vi "Adjust Dashboard Window_NO_RESIZE.vi"(6 "Sizing Refnums":T1, 9 "Size Constraints":cluster{"min tab width":i32, "w/h":dbl}, 10 "VI":refnum<vi>, 11 "WIn Mode":refnum<notifier>) -> ()   [LabVIEW 2023]
panel:
  in  "Str Refnum":refnum<vi>
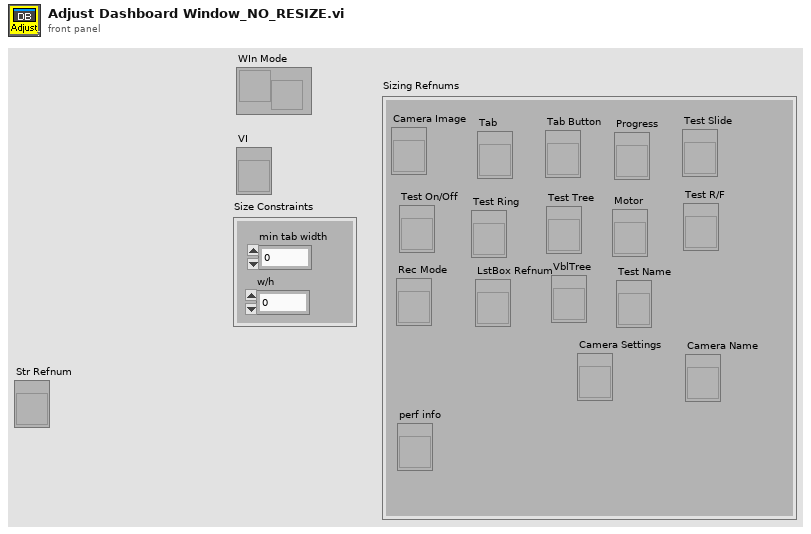
[diagram p1: front panel]
types:
  T1 = cluster{"Camera Image":refnum<vi>, "Tab":refnum<vi>, "Tab Button":refnum<vi>, "Rec Mode":refnum<vi>, "Test Slide":refnum<vi>, "Test On/Off":refnum<vi>, "Test Ring":refnum<vi>, "Test R/F":refnum<vi>, "Test Name":refnum<vi>, "Motor":refnum<vi>, "Progress":refnum<vi>, "LstBox Refnum":refnum<vi>, "Test Tree":refnum<vi>, "VblTree":refnum<vi>, "Camera Settings":refnum<vi>, "Camera Name":refnum<vi>, "perf info":refnum<vi>}
  T2 = typedef "LVRectTypeDef.ctl" = cluster{"Left":i16, "Top":i16, "Right":i16, "Bottom":i16}
  T3 = typedef "LVPointTypeDef.ctl" = cluster{"Horizontal":i16, "Vertical":i16}
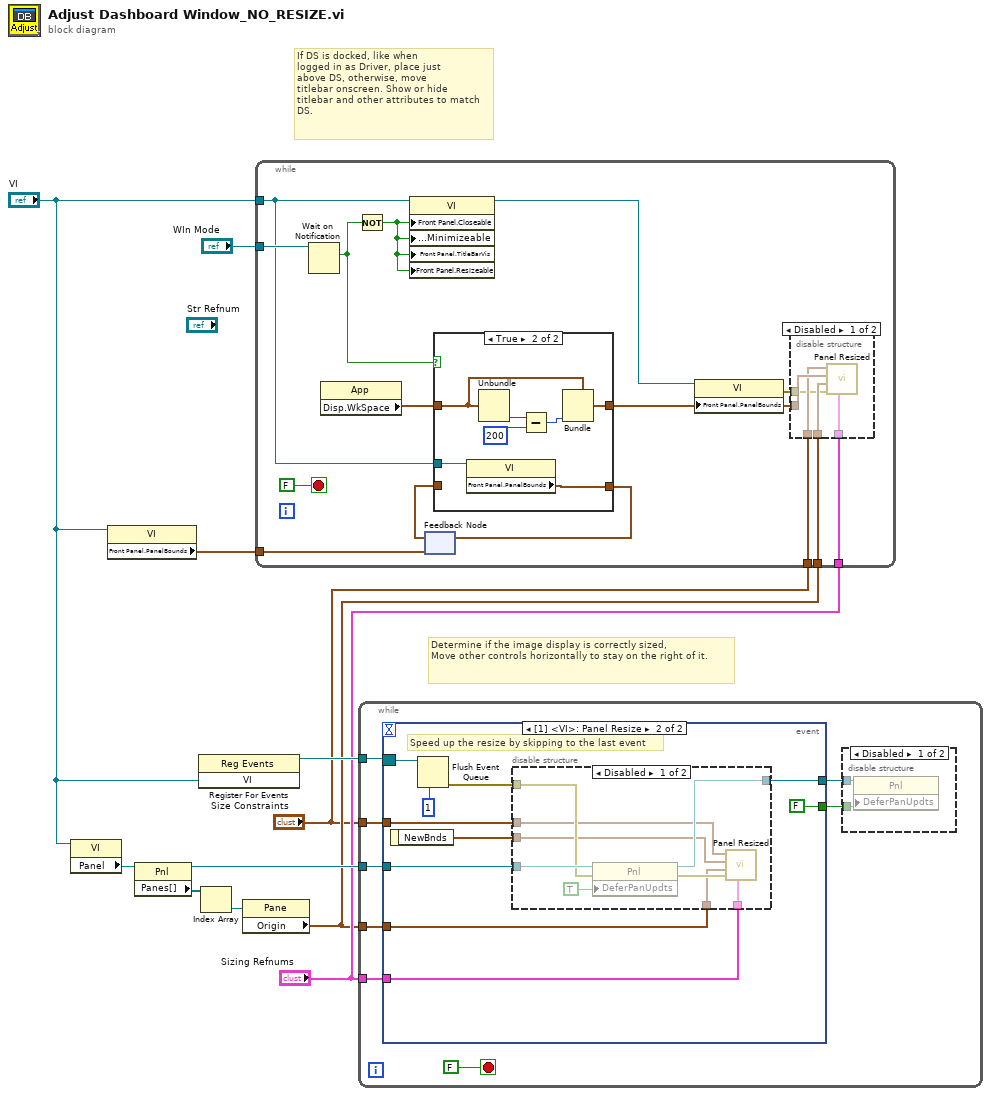
[diagram p0: block diagram]
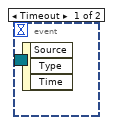
[diagram p3: hidden frame]
diagram:
  # "Determine if the image display is correctly sized,\nMove other controls horizontally to stay on the right of it."
  # "If DS is docked, like when\nlogged in as Driver, place just\nabove DS, otherwise, move\ntitlebar onscreen. Show or hide\ntitlebar and other attributes to match\nDS."
  n1 = property class="VI"(reference="VI") -> ("Panel"=w9:refnum<vi>)  [unwired: 1 in, 2 out]
  n2 = property class="VI"(reference="VI") -> ("Front Panel.PanelBounds"=w2:T2)  [unwired: 1 in, 2 out]
  n3 = property class="Pnl"(reference=w9) -> (reference out=w6:refnum<vi>, "Panes[]"=w8:refnum<vi>[])  [unwired: 1 in, 1 out]
  n4 = register-events("VI") -> (reference out=w10:refnum<event-registration>)  [unwired: 2 in, 1 out]
  n5 = Index Array(array=w8) -> (element=w7:refnum<vi>)  [unwired: 1 in]
  n6 = property class="Pane"(reference=w7) -> ("Origin"=w4:T3)  [unwired: 1 in, 2 out]
  n7 = while {
    tunnel: "WIn Mode" -> [w25]
    tunnel: "VI" -> [w17]
    tunnel: "Sizing Refnums" -> [w22]
    tunnel: w4 -> [w21]
    tunnel: "Size Constraints" -> [w19]
    tunnel: w2 -> [w14]
    stop <- FALSE stop-if-true
    n8 = Wait on Notification(notifier=w25) -> (notification=w18:bool)  [unwired: 3 in, 3 out]
    n9 = property class="App"() -> ("Disp.WkSpace"=w24:T2)  [unwired: 2 in, 2 out]
    n10 = Not(x=w18) -> (.not. x?=w13:bool)
    n11 = property class="VI"(reference=w17, "Front Panel.Closeable"=w13, "Front Panel.Minimizeable"=w13, "Front Panel.TitleBarVis"=w13, "Front Panel.Resizeable"=w13) -> (reference out=w23:refnum<vi>)  [unwired: 1 in, 1 out]
    n12 = feedback #1(w14) -> (w15:T2)
    n13 = case shown="True" w18 {
      tunnel: w24 -> [_ w35]
      tunnel: [w32 w36] -> w20
      tunnel: w17 -> [_ w34]
      tunnel: [w32 w33] -> w16
      tunnel: w15 -> [w32 _]
      frame False {
      }
      frame True {
        n14 = property class="VI"(reference=w34) -> ("Front Panel.PanelBounds"=w33:T2)  [unwired: 1 in, 2 out]
        n15 = Unbundle(w35) -> ("Bottom"=w39:i16)  [unwired: 3 out]
        n16 = Subtract(x=w39, y=200) -> (x-y=w37:i32)
        n17 = Bundle(cluster=w35, "Bottom"=w37) -> (w36:T2)  [unwired: 3 out]
      }
    }
    n18 = feedback-in #1(w16) -> ()
    n19 = property class="VI"(reference=w23, "Front Panel.PanelBounds"=w20) -> (error out=w12:errorcluster)  [unwired: 1 in, 1 out]
    n20 = disable-structure shown="Disabled" {
      disable-tunnel: w22 -> [w31 _]
      disable-tunnel: w21 -> [w30 _]
      disable-tunnel: w20 -> [w29 _]
      disable-tunnel: w19 -> [w28 _]
      disable-tunnel: w12 -> [w27 _]
      frame Disabled {
        n21 = call "Panel Resized.vi"("Sizing Refnums"=w31, "error in (no error)"=w27, "Origin"=w30, "NewBnds"=w29, "Size Constraints"=w28) -> ()  [unwired: 6 in, 1 out]
      }
      frame Enabled {
      }
    }
  }
  n22 = while {
    tunnel: w10 -> [w46]
    tunnel: "Sizing Refnums" -> [w45]
    tunnel: "Size Constraints" -> [w44]
    tunnel: w4 -> [w43]
    tunnel: w6 -> [w42]
    stop <- FALSE stop-if-true
    n23 = event shown="[1] <VI>: Panel Resize" {
      selector: w46 -> [_ w57]
      dyn-events: _ -> [_ _]
      timeout: _ -> [_ _]
      tunnel: w45 -> [_ w50]
      tunnel: w44 -> [_ w53]
      tunnel: w43 -> [_ w51]
      tunnel: w42 -> [_ w59]
      tunnel: [_ FALSE ("Defer Panel Updates")] -> w41
      tunnel: [_ w54] -> w40
      event Timeout {
        n24 = event-data() -> ()  [unwired: 1 in, 3 out]
      }
      event Panel Resize {
        # "Speed up the resize by skipping to the last event"
        n25 = event-data() -> ("NewBnds"=w52:T2)  [unwired: 1 in]
        n26 = Flush Event Queue(0:w57, 5:1 ("keep most recent")) -> (11:w55:errorcluster)  [unwired: 4 in, 2 out]
        n27 = disable-structure shown="Disabled" {
          disable-tunnel: w59 -> [w68 _]
          disable-tunnel: w55 -> [w66 _]
          disable-tunnel: [w65 _] -> w54
          disable-tunnel: w53 -> [w63 _]
          disable-tunnel: w52 -> [w62 _]
          disable-tunnel: w51 -> [w61 _]
          disable-tunnel: w50 -> [w60 _]
          frame Disabled {
            n28 = property class="Pnl"(reference=w68, error in=w66, "DeferPanUpdts"=TRUE ("Defer Panel Updates")) -> (reference out=w65:refnum<vi>, error out=w64:errorcluster)
            n29 = call "Panel Resized.vi"("Sizing Refnums"=w60, "error in (no error)"=w64, "Origin"=w61, "NewBnds"=w62, "Size Constraints"=w63) -> ()  [unwired: 6 in, 1 out]
          }
          frame Enabled {
          }
        }
      }
    }
    n30 = disable-structure shown="Disabled" {
      disable-tunnel: w41 -> [w49 _]
      disable-tunnel: w40 -> [w48 _]
      frame Disabled {
        n31 = property class="Pnl"(reference=w48, "DeferPanUpdts"=w49) -> ()  [unwired: 1 in, 2 out]
      }
      frame Enabled {
      }
    }
  }
